vi "Read WH Initiale Value.vi"(8 "error in (no error)":errorcluster, 11 "Universal Card in":refnum<class "Universal Card.lvclass">) -> (0 "error out":errorcluster, 2 "WH Initiale Value":dbl, 3 "Universal Card out":refnum<class "Universal Card.lvclass">)   [LabVIEW 2014, in "Universal Power Meter.lvlib" / "Universal Card.lvclass"]
uses:
  Universal Card.lvclass
  Universal Card.lvclass/Universal Card.ctl
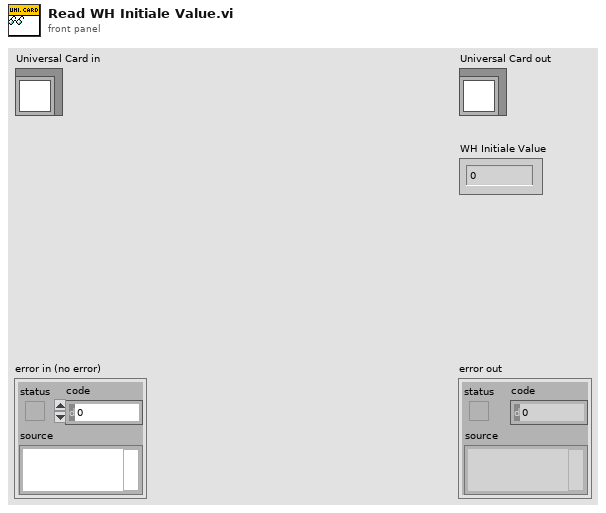
[diagram p1: front panel]
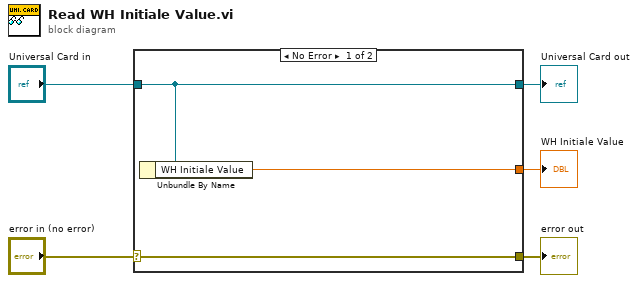
[diagram p0: block diagram]
diagram:
  n1 = case shown="No Error" "error in (no error)" {
    selector: "error in (no error)" -> [w8 w9]
    tunnel: [w8 w9] -> w4
    tunnel: [w7 w10] -> w2
    tunnel: "Universal Card in" -> [w7 w10]
    tunnel: [w6 _] -> w1
    frame No Error {
      n2 = Unbundle By Name(w7) -> ("WH Initiale Value"=w6:dbl)
    }
    frame Error {
    }
  }
  "error out" <- w4
  "Universal Card out" <- w2
  "WH Initiale Value" <- w1
